vi "Programa_robot_final.vi"() -> ()   [LabVIEW 2019]
uses:
  <vilib>/Instr/_visa.llb/VISA Configure Serial Port (Instr).vi
  <vilib>/regexp/Match Regular Expression.xnode
panel:
  in  "?":bool=TRUE
  in  "?":bool
  out "Boolean":bool
  in  "Cerrar socket":bool
  in  "Abrir socket":bool
  out "Error_QR":bool
  in  "Interruptor Error":bool
  in  "stop socket 2":bool
  out "Bytes at port 3":u32=1
  in  "IN y":string(combo)="00"
  in  "IN x":string(combo)="00"
  in  "NOK y":string(combo)="00"
  in  "NOK x":string(combo)="00"
  in  "OK y":string(combo)="00"
  in  "OK x":string(combo)="00"
  in  "Operator's name":string(combo)="Juan Rodríguez"
  in  "?":bool
  in  "Fichero de registro":path=path "C:/Trabajo/Caracterizacion ADCs/Registro_DACs_buenos.txt"
  in  "Config File":path=path "C:/Trabajo/Test Asic Javi_2021/Origen Socket SERVO_PCB_BUENO_v5 (muchos asics)/CONFIG/configuracion_robot_CTAV2022A.test"
  in  "Path Out Report":path=path "C:/Trabajo/Caracterizacion ADCs/PruebasDACs_buenos"
  out "Datos_QR":string
  in  "stop socket":bool
  out "Bytes at port 1":u32
  in  "Enviar":bool
  out "Iteraciones":i32
  out "Lectura buffer":string="1"
  in  "Delay (ms)":dbl=1.0 min=1.0 max=9.0 step=1.0
  out "Bytes at port 2":u32=1
  out "message":string=" INSTRUCTIONS:\r\rNormal Use:  When using subVIs that incorporate the error in/error out (or error I/O) structure, place this handler where you want to inform the user of an error, typically at the end of the I/O data path, as the last action of the program.  If the error in error? is ERROR, the handler creates a message describing the error and its source.  If the type of dialog = 1 (default), the message is displayed to the user, who can only acknowedge it.  If the type = 2, the user can acknowledge the message or abort execution; aborting a program with active I/O is not recommended.  If the type = 0, no message is displayed; this is used to process the error programmatically, and the error out cluster elements are wired to individual terminals for that reason.  \r\rOther Use:\n\r\nlocal testing.  To test the error code of a subVI or function that does not have the error I/O structure, you can wire its error code and a source string to the local error code and error source inputs.  If error in error? indicates no error and error code is not equal to 0, the local code and source are substituted for the error in values, and error? is set TRUE (ERROR)."
  in  "Interruptor":bool=TRUE
  in  "stop":bool
  # "Funcionamiento: en la primera iteración, el efector se desplaza desde el origen hasta la celda\nintroducida, hace una pausa, va a la posición del socket (0,0), hace otra pausa, va a la celda\nde salida y vuelve al origen. En las iteraciones siguientes hará lo mismo pero recorriendo las\nceldas de la bandeja sucesivamente. Que el desplazamiento se produzca hacia una celda de\nla bandeja OK o de la bandeja NOK depende de la salidad del programa de test de Asics."
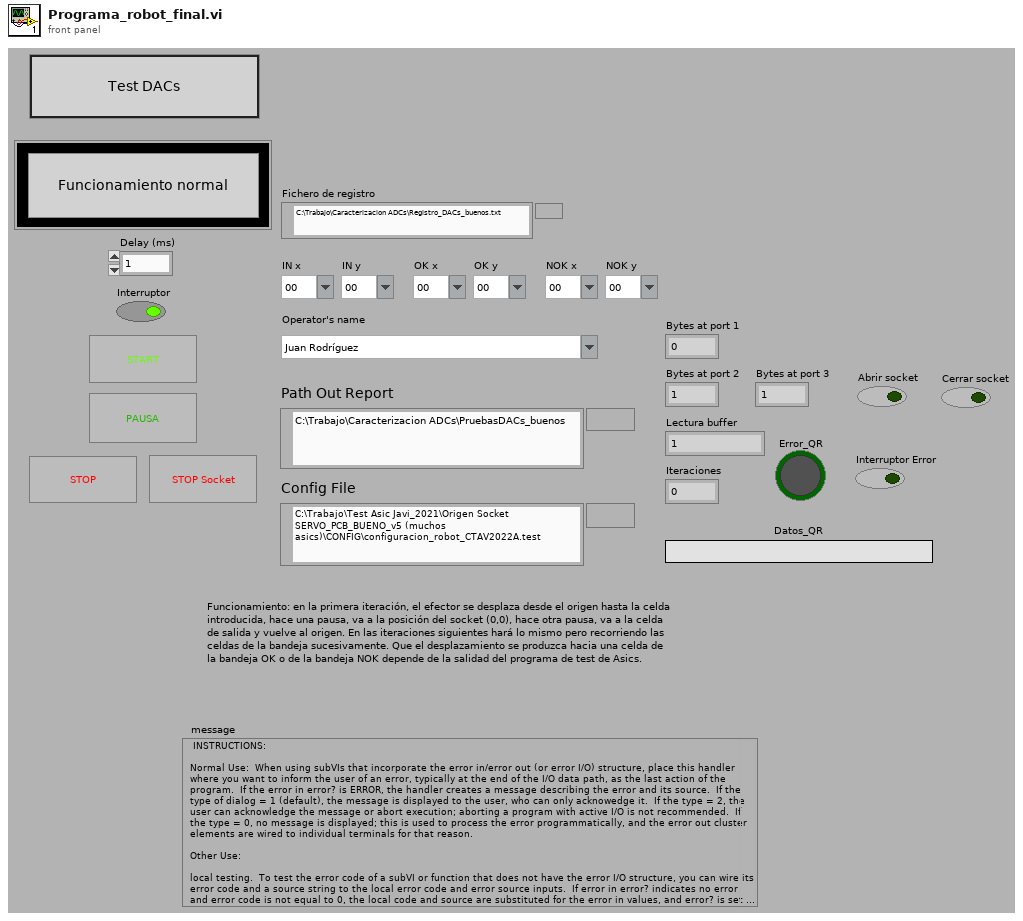
[diagram p1: front panel]
types:
  T1 = enum16{"open", "replace", "create", "open or create", "replace or create", "replace or create with confirmation"}
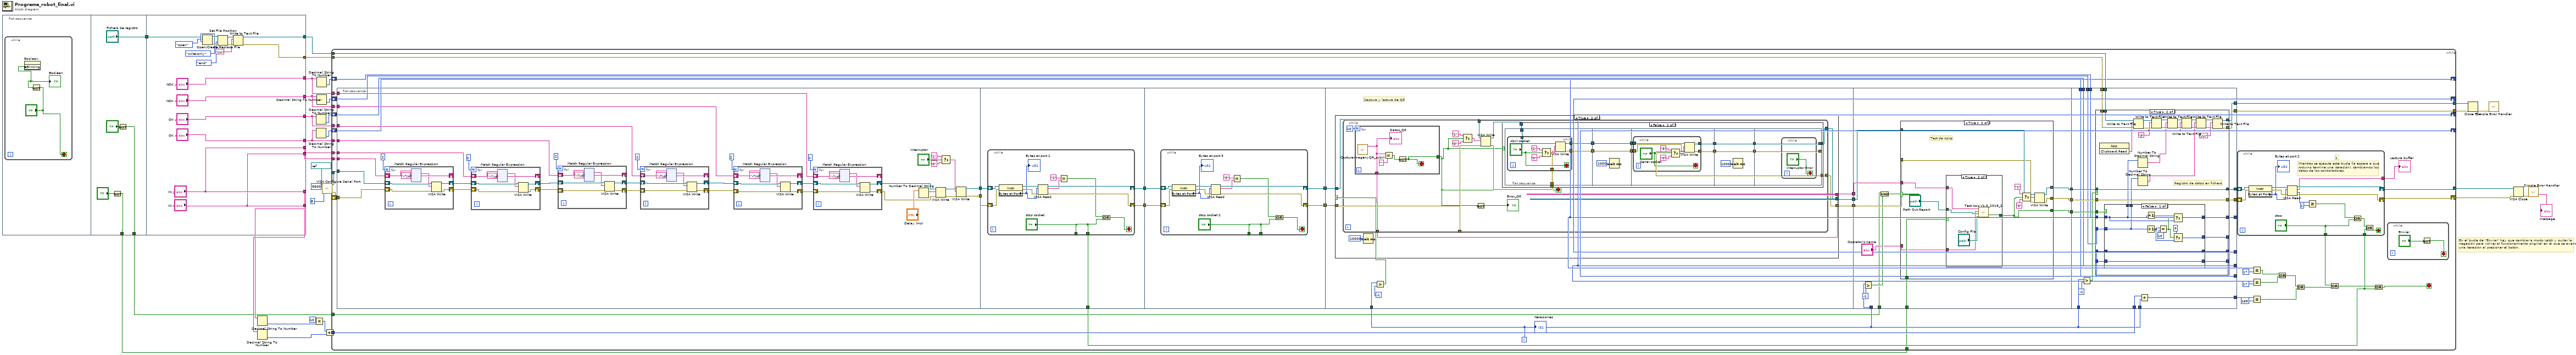
[diagram p0: block diagram]
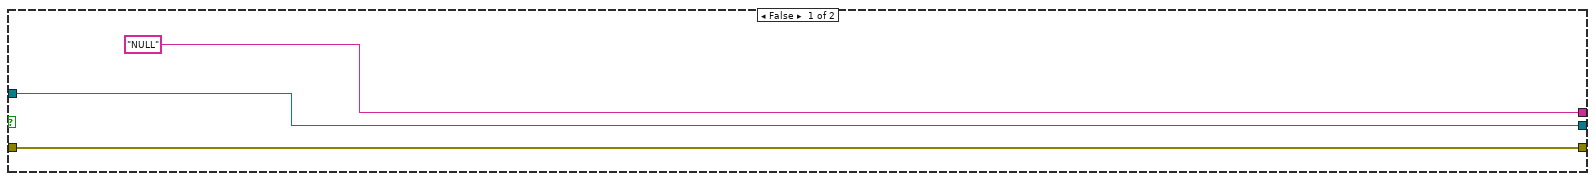
[diagram p2: hidden frame]
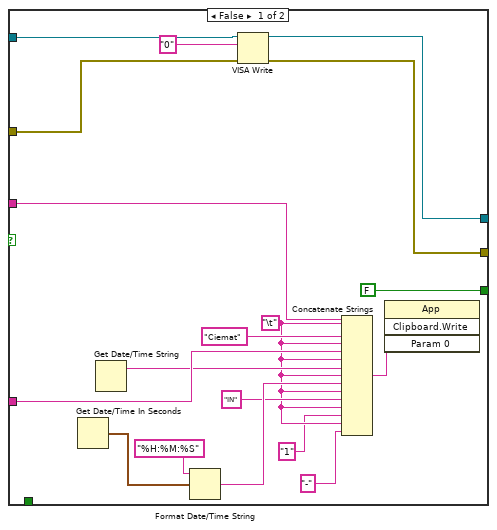
[diagram p4: hidden frame]
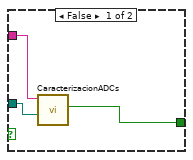
[diagram p5: hidden frame]
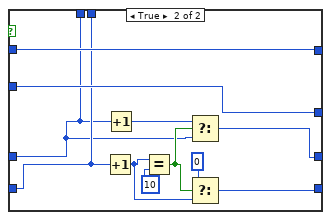
[diagram p7: hidden frame]
diagram:
  # "En el bucle de \"Enviar\" hay que cambiar a modo Latch y quitar la\nnegación para volver al funcionamiento original en el que se avanza\nuna iteración al presionar el botón."
  n1 = flat-sequence {
    tunnel: [w40] -> w3
    tunnel: [w39] -> w2
    tunnel: ["Fichero de registro"] -> w1
    tunnel: ["NOK y"] -> w18
    tunnel: ["NOK x"] -> w17
    tunnel: ["OK y"] -> w16
    tunnel: ["OK x"] -> w15
    tunnel: ["IN y"] -> w14
    tunnel: ["IN x"] -> w13
    tunnel: [w43] -> w12
    tunnel: [w44] -> w11
    tunnel: ["IN y"] -> w10
    tunnel: ["IN x"] -> w9
    tunnel: w1 -> [w42]
    frame #0 {
      n2 = while {
        stop <- "?" stop-if-true
        n3 = Not(x="?") -> (.not. x?=w35:bool)
        "Boolean" <- w35
        n4 = property on="Boolean" class="Bool (strict)"("Blinking"=w35) -> ()  [unwired: 2 in, 2 out]
      }
    }
    frame #1 {
      n5 = Not(x="?") -> (.not. x?=w39:bool)
      n6 = Not(x="?") -> (.not. x?=w40:bool)
    }
    frame #2 {
      n7 = Open/Create/Replace File(file path (use dialog)=w42, operation (0:open)=T1."open", access (0:read/write)=enum16{"read/write", "read-only", "write-only"}."write-only") -> (refnum out=w55:refnum<file>, error out=w57:errorcluster)  [unwired: 3 in, 1 out]
      n8 = Set File Position(refnum=w55, from (0:start)=enum16{"start", "end", "current"}."end", error in=w57) -> (refnum out=w56:refnum<file>, error out=w58:errorcluster)  [unwired: 1 in]
      n9 = Write to Text File(file (use dialog)=w56, text="\r\n", error in=w58) -> (refnum out=w44:refnum<file>, error out=w43:errorcluster)  [unwired: 1 in, 1 out]
    }
  }
  n10 = Decimal String To Number(string=w10) -> (number=w8:i32)  [unwired: 2 in, 1 out]
  n11 = Decimal String To Number(string=w9) -> (number=w5:i32)  [unwired: 2 in, 1 out]
  n12 = Multiply(x=10, y=w8) -> (x*y=w6:i32)
  n13 = Decimal String To Number(string=w16) -> (number=w20:i32)  [unwired: 2 in, 1 out]
  n14 = Decimal String To Number(string=w15) -> (number=w19:i32)  [unwired: 2 in, 1 out]
  n15 = Decimal String To Number(string=w18) -> (number=w22:i32)  [unwired: 2 in, 1 out]
  n16 = Decimal String To Number(string=w17) -> (number=w21:i32)  [unwired: 2 in, 1 out]
  n17 = call-poly "VISA Configure Serial Port"("VISA resource name"=refnum<visa-resource-name> "COM9", "baud rate (9600)"=u32 9600, "data bits (8)"=u16 8) -> ("VISA resource name out"=w26:refnum<visa-resource-name>, "error out"=w29:errorcluster)  [unwired: 11 in]
  n18 = Add(x=w6, y=w5) -> (x+y=w4:i32)
  n19 = while {
    shift-right: [w110] -> w27
    shift-left: w29 -> [w112]
    tunnel: w26 -> [w108]
    tunnel: [w111] -> w28
    tunnel: w11 -> [w101]
    tunnel: [w100] -> w25
    tunnel: w12 -> [w99]
    tunnel: [w98] -> w24
    tunnel: w13 -> [w96]
    tunnel: w14 -> [w95]
    tunnel: w15 -> [w94]
    tunnel: w16 -> [w93]
    tunnel: w17 -> [w92]
    tunnel: w18 -> [w91]
    shift-right: [w84] -> _
    shift-left: w22 -> [w90]
    shift-right: [w86] -> _
    shift-left: w21 -> [w89]
    shift-right: [w82] -> _
    shift-left: w20 -> [w88]
    shift-right: [w85] -> _
    shift-left: w19 -> [w87]
    tunnel: w4 -> [w78]
    tunnel: w3 -> [w60]
    tunnel: w2 -> [w59]
    i -> [w61]
    stop <- w70 stop-if-true
    n20 = flat-sequence {
      tunnel: w112 -> [w148]
      tunnel: w108 -> [w137]
      tunnel: [w139] -> w107
      tunnel: [w138] -> w106
      tunnel: w96 -> [w118]
      tunnel: w95 -> [w117]
      tunnel: w94 -> [w116]
      tunnel: w93 -> [w115]
      tunnel: w92 -> [w114]
      tunnel: w91 -> [w113]
      tunnel: w107 -> [w885]
      tunnel: w106 -> [w884]
      tunnel: [w883] -> w68
      tunnel: [w882] -> w66
      tunnel: [w881] -> w69
      tunnel: w68 -> [w901]
      tunnel: [w899] -> w67
      tunnel: w66 -> [w900]
      tunnel: [w898] -> w65
      tunnel: w67 -> [w919]
      tunnel: w65 -> [w918]
      tunnel: w61 -> [w920]
      tunnel: [w916] -> w64
      tunnel: [w915] -> w63
      tunnel: [w914] -> w62
      tunnel: w61 -> [w1005]
      tunnel: [w1007] -> w104
      tunnel: [w1006] -> w103
      tunnel: [w1003] -> w97
      tunnel: w64 -> [w1002]
      tunnel: w63 -> [w1001]
      tunnel: w62 -> [w1000]
      tunnel: w60 -> [w997]
      tunnel: w59 -> [w996]
      tunnel: [w1062] -> w102
      tunnel: [w1064] -> w105
      tunnel: w104 -> [w1063]
      tunnel: w103 -> [w1061]
      tunnel: w101 -> [w1068]
      tunnel: [w1067] -> w100
      tunnel: w99 -> [w1066]
      tunnel: [w1065] -> w98
      tunnel: w61 -> [w1058]
      tunnel: w97 -> [w1057]
      tunnel: w90 -> [w1053]
      tunnel: w89 -> [w1056]
      tunnel: w88 -> [w1055]
      tunnel: w87 -> [w1054]
      tunnel: [w1052] -> w84
      tunnel: [w1051] -> w86
      tunnel: [w1050] -> w82
      tunnel: [w1049] -> w85
      tunnel: w78 -> [w1048]
      tunnel: w61 -> [w1047]
      tunnel: [w1046] -> w77
      frame #0 {
        n21 = for {
          N: 2 -> [_]
          shift-right: [w760] -> _
          shift-left: w118 -> [w765]
          shift-right: [w763] -> w134
          shift-left: w137 -> [w764]
          shift-right: [w761] -> w133
          shift-left: w148 -> [w762]
          n22 = xnode "Match Regular Expression"("input string"=w765, "regular expression"="-?\\d") -> ("whole match"=w759:string, "after match"=w760:string)  [unwired: 4 in, 3 out]
          n23 = VISA Write(VISA resource name=w764, write buffer=w759, error in (no error)=w762) -> (VISA resource name out=w763:refnum<visa-resource-name>, error out=w761:errorcluster)  [unwired: 1 out]
        }
        n24 = for {
          N: 2 -> [_]
          shift-right: [w638] -> _
          shift-left: w117 -> [w643]
          shift-right: [w641] -> w128
          shift-left: w134 -> [w642]
          shift-right: [w639] -> w127
          shift-left: w133 -> [w640]
          n25 = xnode "Match Regular Expression"("input string"=w643, "regular expression"="-?\\d") -> ("whole match"=w637:string, "after match"=w638:string)  [unwired: 4 in, 3 out]
          n26 = VISA Write(VISA resource name=w642, write buffer=w637, error in (no error)=w640) -> (VISA resource name out=w641:refnum<visa-resource-name>, error out=w639:errorcluster)  [unwired: 1 out]
        }
        n27 = for {
          N: 2 -> [_]
          shift-right: [w516] -> _
          shift-left: w116 -> [w521]
          shift-right: [w519] -> w130
          shift-left: w128 -> [w520]
          shift-right: [w517] -> w129
          shift-left: w127 -> [w518]
          n28 = xnode "Match Regular Expression"("input string"=w521, "regular expression"="-?\\d") -> ("whole match"=w515:string, "after match"=w516:string)  [unwired: 4 in, 3 out]
          n29 = VISA Write(VISA resource name=w520, write buffer=w515, error in (no error)=w518) -> (VISA resource name out=w519:refnum<visa-resource-name>, error out=w517:errorcluster)  [unwired: 1 out]
        }
        n30 = for {
          N: 2 -> [_]
          shift-right: [w394] -> _
          shift-left: w115 -> [w399]
          shift-right: [w397] -> w122
          shift-left: w130 -> [w398]
          shift-right: [w395] -> w121
          shift-left: w129 -> [w396]
          n31 = xnode "Match Regular Expression"("input string"=w399, "regular expression"="-?\\d") -> ("whole match"=w393:string, "after match"=w394:string)  [unwired: 4 in, 3 out]
          n32 = VISA Write(VISA resource name=w398, write buffer=w393, error in (no error)=w396) -> (VISA resource name out=w397:refnum<visa-resource-name>, error out=w395:errorcluster)  [unwired: 1 out]
        }
        n33 = for {
          N: 2 -> [_]
          shift-right: [w272] -> _
          shift-left: w114 -> [w277]
          shift-right: [w275] -> w124
          shift-left: w122 -> [w276]
          shift-right: [w273] -> w123
          shift-left: w121 -> [w274]
          n34 = xnode "Match Regular Expression"("input string"=w277, "regular expression"="-?\\d") -> ("whole match"=w271:string, "after match"=w272:string)  [unwired: 4 in, 3 out]
          n35 = VISA Write(VISA resource name=w276, write buffer=w271, error in (no error)=w274) -> (VISA resource name out=w275:refnum<visa-resource-name>, error out=w273:errorcluster)  [unwired: 1 out]
        }
        n36 = for {
          N: 2 -> [_]
          shift-right: [w150] -> _
          shift-left: w113 -> [w155]
          shift-right: [w153] -> w120
          shift-left: w124 -> [w154]
          shift-right: [w151] -> w119
          shift-left: w123 -> [w152]
          n37 = xnode "Match Regular Expression"("input string"=w155, "regular expression"="-?\\d") -> ("whole match"=w149:string, "after match"=w150:string)  [unwired: 4 in, 3 out]
          n38 = VISA Write(VISA resource name=w154, write buffer=w149, error in (no error)=w152) -> (VISA resource name out=w153:refnum<visa-resource-name>, error out=w151:errorcluster)  [unwired: 1 out]
        }
        n39 = Number To Decimal String(number="Delay (ms)") -> (decimal integer string=w142:string)  [unwired: 1 in]
        n40 = VISA Write(VISA resource name=w120, write buffer=w142, error in (no error)=w119) -> (VISA resource name out=w144:refnum<visa-resource-name>, error out=w143:errorcluster)  [unwired: 1 out]
        n41 = Select(t="1" ("write buffer"), s="Interruptor", f="0" ("write buffer")) -> (s? t:f=w140:string)
        n42 = VISA Write(VISA resource name=w144, write buffer=w140, error in (no error)=w143) -> (VISA resource name out=w139:refnum<visa-resource-name>, error out=w138:errorcluster)  [unwired: 1 out]
      }
      frame #1 {
        n43 = while {
          shift-right: [w891] -> w882
          shift-left: w884 -> [w896]
          tunnel: ["stop socket"] -> _
          shift-right: [w892] -> w883
          shift-left: w885 -> [w897]
          tunnel: ["stop socket"] -> w881
          stop <- w887 stop-if-true
          n44 = property class="Instr"(reference=w897, error in=w896) -> (reference out=w895:refnum<visa-resource-name>, error out=w894:errorcluster, "Bytes at Port"=w893:u32)
          "Bytes at port 1" <- w893
          n45 = VISA Read(VISA resource name=w895, byte count=w893, error in (no error)=w894) -> (VISA resource name out=w892:refnum<visa-resource-name>, read buffer=w890:string, error out=w891:errorcluster)  [unwired: 1 out]
          n46 = Equal?(x="2", y=w890) -> (x = y?=w888:bool)
          n47 = Or(x=w888, y="stop socket") -> (x .or. y?=w887:bool)
        }
      }
      frame #2 {
        n48 = while {
          shift-right: [w907] -> w898
          shift-left: w900 -> [w912]
          tunnel: ["stop socket 2"] -> _
          shift-right: [w908] -> w899
          shift-left: w901 -> [w913]
          tunnel: ["stop socket 2"] -> _
          stop <- w903 stop-if-true
          n49 = property class="Instr"(reference=w913, error in=w912) -> (reference out=w911:refnum<visa-resource-name>, error out=w910:errorcluster, "Bytes at Port"=w909:u32)
          "Bytes at port 3" <- w909
          n50 = VISA Read(VISA resource name=w911, byte count=w909, error in (no error)=w910) -> (VISA resource name out=w908:refnum<visa-resource-name>, read buffer=w906:string, error out=w907:errorcluster)  [unwired: 1 out]
          n51 = Equal?(x="3", y=w906) -> (x = y?=w904:bool)
          n52 = Or(x=w904, y="stop socket 2") -> (x .or. y?=w903:bool)
        }
      }
      frame #3 {
        # "Captura y lectura de QR"
        n53 = Greater?(x=w920, y=-1) -> (0:w917:bool)
        n54 = case shown="True" w917 {
          tunnel: [w924 w927] -> w914
          tunnel: w919 -> [w924 w928]
          tunnel: [w923 w926] -> w916
          tunnel: w918 -> [w923 w925]
          tunnel: ["NULL" ("Datos_QR") w929] -> w915
          frame False {
          }
          frame True {
            n55 = while {
              tunnel: [w943] -> w929
              tunnel: w928 -> [w941]
              tunnel: [w937] -> w927
              tunnel: [w936] -> w926
              tunnel: w925 -> [w934]
              stop <- w931 stop-if-true
              n56 = for {
                N: 10 -> [_]
                tunnel: [w991] -> w943
                tunnel: [w992] -> w931
                stop <- w992 stop-if-true
                n57 = call "CapturaImagenyQR_subVI.vi"() -> ("Datos_QR"=w991:string)  [unwired: 11 in]
                "Datos_QR" <- w991
                n58 = Equal?(x=w991, y="" ("Datos_QR")) -> (x = y?=w993:bool)
                n59 = Not(x=w993) -> (.not. x?=w992:bool)
              }
              n60 = Select(t="1" ("write buffer"), s=w931, f="0" ("write buffer")) -> (s? t:f=w938:string)
              n61 = Not(x=w931) -> (.not. x?=→"Error_QR":bool)
              n62 = VISA Write(VISA resource name=w941, write buffer=w938, error in (no error)=w934) -> (VISA resource name out=w935:refnum<visa-resource-name>, error out=w933:errorcluster)  [unwired: 1 out]
              n63 = case shown="False" w931 {
                tunnel: w935 -> [w955 w990]
                tunnel: w933 -> [w954 w989]
                tunnel: [w953 w990] -> w937
                tunnel: [w952 w989] -> w936
                frame False {
                  n64 = flat-sequence {
                    tunnel: w955 -> [w959]
                    tunnel: [w958] -> w951
                    tunnel: [w957] -> w949
                    tunnel: w954 -> [w956]
                    tunnel: w951 -> [w970]
                    tunnel: [w970] -> w950
                    tunnel: w949 -> [w969]
                    tunnel: [w969] -> w948
                    tunnel: w950 -> [w974]
                    tunnel: w948 -> [w973]
                    tunnel: [w972] -> w947
                    tunnel: [w971] -> w945
                    tunnel: w947 -> [w985]
                    tunnel: [w985] -> w946
                    tunnel: w945 -> [w984]
                    tunnel: [w984] -> w944
                    tunnel: [w986] -> w952
                    tunnel: [w987] -> w953
                    tunnel: w946 -> [w987]
                    tunnel: w944 -> [w986]
                    frame #0 {
                      n65 = while {
                        tunnel: w959 -> [w967]
                        tunnel: [w962] -> w958
                        tunnel: [w961] -> w957
                        tunnel: w956 -> [w960]
                        stop <- "Abrir socket" stop-if-true
                        n66 = Select(t="2" ("write buffer"), s="Abrir socket", f="0" ("write buffer")) -> (s? t:f=w964:string)
                        n67 = VISA Write(VISA resource name=w967, write buffer=w964, error in (no error)=w960) -> (VISA resource name out=w962:refnum<visa-resource-name>, error out=w961:errorcluster)  [unwired: 1 out]
                      }
                    }
                    frame #1 {
                      n68 = Wait (ms)(milliseconds to wait=u32 1000) -> ()  [unwired: 1 out]
                    }
                    frame #2 {
                      n69 = while {
                        tunnel: w974 -> [w978]
                        tunnel: w973 -> [w977]
                        tunnel: [w976] -> w972
                        tunnel: [w975] -> w971
                        stop <- "Cerrar socket" stop-if-true
                        n70 = Select(t="3" ("write buffer"), s="Cerrar socket", f="0" ("write buffer")) -> (s? t:f=w980:string)
                        n71 = VISA Write(VISA resource name=w978, write buffer=w980, error in (no error)=w977) -> (VISA resource name out=w976:refnum<visa-resource-name>, error out=w975:errorcluster)  [unwired: 1 out]
                      }
                    }
                    frame #3 {
                      n72 = Wait (ms)(milliseconds to wait=u32 1000) -> ()  [unwired: 1 out]
                    }
                    frame #4 {
                      n73 = while {
                        stop <- "Interruptor Error" stop-if-true
                      }
                    }
                  }
                }
                frame True {
                }
              }
            }
            n74 = Wait (ms)(milliseconds to wait=u32 10000) -> ()  [unwired: 1 out]
          }
        }
      }
      frame #4 {
        n75 = Greater?(x=w1005, y=-1) -> (0:w999:bool)
        n76 = And(x=w997, y=w999) -> (x .and. y?=w998:bool)
        n77 = case shown="True" w998 {
          tunnel: w1000 -> [w1023 w1034]
          tunnel: w1002 -> [w1022 w1033]
          tunnel: [w1021 w1032] -> w1007
          tunnel: [w1020 w1031] -> w1006
          tunnel: w1001 -> [w1016 w1030]
          tunnel: [FALSE ("Boolean") w1028] -> w1003
          tunnel: "Operator's name" -> [w1014 w1026]
          tunnel: w996 -> [_ w1027]
          frame False {
            w1010 = "\t"
            n78 = Get Date/Time In Seconds() -> (seconds since 1Jan1904=w1018:timestamp)
            n79 = Get Date/Time String() -> (date string=w1013:string)  [unwired: 3 in, 1 out]
            n80 = Format Date/Time String(time format string (%c)="%H:%M:%S", seconds (now)=w1018) -> (date/time string=w1012:string)  [unwired: 1 in]
            n81 = VISA Write(VISA resource name=w1023, write buffer="0", error in (no error)=w1022) -> (VISA resource name out=w1021:refnum<visa-resource-name>, error out=w1020:errorcluster)  [unwired: 1 out]
            n82 = Concatenate Strings(w1016, w1010, "Ciemat", w1010, w1014, w1010, w1013, w1010, w1012, w1010, "IN", w1010, "1", w1010, "-") -> (w1019:string)
            n83 = invoke class="App" method="Clipboard.Write"("Param 0"=w1019) -> ()  [unwired: 3 in, 4 out]
          }
          frame True {
            # "Test de Asics"
            n84 = case shown="True" w1027 {
              tunnel: w1030 -> [w1040 w1042]
              tunnel: "Path Out Report" -> [w1039 w1045]
              tunnel: [w1038 w1044] -> w1028
              tunnel: w1026 -> [_ w1041]
              frame False {
                n85 = call "CaracterizacionADCs.vi"("QR code"=w1040, "Path Out Report"=w1039) -> ("OK/NOK"=w1038:bool)  [unwired: 7 in]
              }
              frame True {
                n86 = call "Test Asic V1.0_2019_2.vi"("Config File"="Config File", "Path Out Report"=w1045, "Operator's Name"=w1041, "ASIC'S Number"=w1042) -> ("OK, Fault 2"=w1044:bool)  [unwired: 1 in]
              }
            }
            n87 = Select(t="1" ("write buffer"), s=w1028, f="0" ("write buffer")) -> (s? t:f=w1035:string)
            n88 = VISA Write(VISA resource name=w1034, write buffer=w1035, error in (no error)=w1033) -> (VISA resource name out=w1032:refnum<visa-resource-name>, error out=w1031:errorcluster)  [unwired: 1 out]
          }
        }
      }
      frame #5 {
        n89 = Greater?(x=w1058, y=-1) -> (0:w1059:bool)
        n90 = case shown="True" w1059 {
          tunnel: w1068 -> [w1074 w1107]
          tunnel: [w1074 w1106] -> w1067
          tunnel: w1066 -> [w1073 w1105]
          tunnel: [w1073 w1104] -> w1065
          tunnel: [w1076 w1103] -> w1064
          tunnel: w1063 -> [w1076 w1103]
          tunnel: [w1075 w1102] -> w1062
          tunnel: w1061 -> [w1075 w1102]
          tunnel: w1057 -> [_ w1100]
          tunnel: w1053 -> [w1072 w1099]
          tunnel: w1056 -> [w1071 w1098]
          tunnel: w1055 -> [w1070 w1097]
          tunnel: w1054 -> [w1069 w1096]
          tunnel: [w1072 w1095] -> w1052
          tunnel: [w1071 w1094] -> w1051
          tunnel: [w1070 w1093] -> w1050
          tunnel: [w1069 w1092] -> w1049
          frame False {
          }
          frame True {
            w1079 = "\t"
            # "Registro de datos en fichero"
            n91 = invoke class="App" method="Clipboard.Read"() -> ("Read Clipbrd"=w1101:string)  [unwired: 3 in, 2 out]
            n92 = case shown="False" w1100 {
              tunnel: w1099 -> [w1110 w1123]
              tunnel: w1098 -> [w1109 w1122]
              tunnel: w1097 -> [w1112 w1120]
              tunnel: w1096 -> [w1111 w1121]
              tunnel: [w1114 w1123] -> w1095
              tunnel: [w1113 w1122] -> w1094
              tunnel: [w1112 w1125] -> w1093
              tunnel: [w1111 w1124] -> w1092
              tunnel: [w1110 w1120] -> w1091
              tunnel: [w1109 w1121] -> w1090
              frame False {
                n93 = Increment(x=w1109) -> (x+1=w1118:i32)
                n94 = Increment(x=w1110) -> (x+1=w1115:i32)
                n95 = Equal?(x=w1118, y=10) -> (x = y?=w1116:bool)
                n96 = Select(t=w1115, s=w1116, f=w1110) -> (s? t:f=w1114:i32)
                n97 = Select(t=0, s=w1116, f=w1118) -> (s? t:f=w1113:i32)
              }
              frame True {
                n98 = Increment(x=w1121) -> (x+1=w1129:i32)
                n99 = Increment(x=w1120) -> (x+1=w1126:i32)
                n100 = Equal?(x=w1129, y=10) -> (x = y?=w1127:bool)
                n101 = Select(t=w1126, s=w1127, f=w1120) -> (s? t:f=w1125:i32)
                n102 = Select(t=0, s=w1127, f=w1129) -> (s? t:f=w1124:i32)
              }
            }
            n103 = Write to Text File(file (use dialog)=w1107, text=w1101, error in=w1105) -> (refnum out=w1088:refnum<file>, error out=w1089:errorcluster)  [unwired: 1 in, 1 out]
            n104 = Number To Decimal String(number=w1091) -> (decimal integer string=w1078:string)  [unwired: 1 in]
            n105 = Number To Decimal String(number=w1090) -> (decimal integer string=w1077:string)  [unwired: 1 in]
            n106 = Write to Text File(file (use dialog)=w1088, text=w1079, error in=w1089) -> (refnum out=w1086:refnum<file>, error out=w1087:errorcluster)  [unwired: 1 in, 1 out]
            n107 = Write to Text File(file (use dialog)=w1086, text=w1078, error in=w1087) -> (refnum out=w1083:refnum<file>, error out=w1082:errorcluster)  [unwired: 1 in, 1 out]
            n108 = Write to Text File(file (use dialog)=w1083, text=w1079, error in=w1082) -> (refnum out=w1081:refnum<file>, error out=w1080:errorcluster)  [unwired: 1 in, 1 out]
            n109 = Write to Text File(file (use dialog)=w1081, text=w1077, error in=w1080) -> (refnum out=w1085:refnum<file>, error out=w1084:errorcluster)  [unwired: 1 in, 1 out]
            n110 = Write to Text File(file (use dialog)=w1085, text="\r\n", error in=w1084) -> (refnum out=w1106:refnum<file>, error out=w1104:errorcluster)  [unwired: 1 in, 1 out]
          }
        }
        n111 = Add(x=w1048, y=w1047) -> (x+y=w1046:i32)
      }
    }
    n112 = while {
      shift-right: [w1140] -> w110
      shift-left: w102 -> [w1146]
      tunnel: ["stop"] -> w72
      shift-right: [w1141] -> w111
      shift-left: w105 -> [w1147]
      tunnel: [w1136] -> w109
      tunnel: w69 -> [w1133]
      stop <- w1135 stop-if-true
      # "1"
      # "Mientras se ejecuta este bucle (la espera a que\nArduino termine una iteración), cambiamos los\ndatos de los controladores."
      n113 = property class="Instr"(reference=w1147, error in=w1146) -> (reference out=w1144:refnum<visa-resource-name>, error out=w1143:errorcluster, "Bytes at Port"=w1142:u32)
      "Bytes at port 2" <- w1142
      n114 = VISA Read(VISA resource name=w1144, byte count=w1142, error in (no error)=w1143) -> (VISA resource name out=w1141:refnum<visa-resource-name>, read buffer=w1136:string, return count=w1139:u32, error out=w1140:errorcluster)
      n115 = Greater Or Equal?(x=w1139, y=u32 1) -> (x >= y?=w1137:bool)
      n116 = Or(x=w1137, y="stop") -> (x .or. y?=w1134:bool)
      n117 = Or(x=w1134, y=w1133) -> (x .or. y?=w1135:bool)
    }
    "Lectura buffer" <- w109
    n118 = Greater Or Equal?(x=w84, y=17) -> (x >= y?=w80:bool)
    n119 = Greater Or Equal?(x=w82, y=17) -> (x >= y?=w79:bool)
    n120 = Greater Or Equal?(x=w77, y=169) -> (x >= y?=w75:bool)
    n121 = Or(x=w80, y=w79) -> (x .or. y?=w74:bool)
    n122 = Or(x=w74, y=w75) -> (x .or. y?=w73:bool)
    n123 = Or(x=w72, y=w73) -> (x .or. y?=w71:bool)
    n124 = Or(x=w71, y=w69) -> (x .or. y?=w70:bool)
    n125 = while {
      stop <- w1131 stop-if-true
      n126 = Not(x="Enviar") -> (.not. x?=w1131:bool)
    }
    "Iteraciones" <- w61
  }
  n127 = Close File(refnum=w25, error in=w24) -> (error out=w23:errorcluster)  [unwired: 1 out]
  n128 = call <vilib>:"Simple Error Handler.vi"("error in (no error)"=w23) -> ()  [unwired: 4 in, 5 out]
  n129 = VISA Close(VISA resource name=w28, error in (no error)=w27) -> (error out=w33:errorcluster)
  n130 = call <vilib>:"Simple Error Handler.vi"("error in (no error)"=w33) -> ("message"=→"message":string)  [unwired: 4 in, 4 out]
